vi "Get Timestamp Definition.vi"(11 "Timestamp in":refnum<class "Timestamp.lvclass">) -> (2 "Definition":T1)   [LabVIEW 2020, in "Conditu2.lvlib" / "Columns.lvlib" / "Timestamp.lvclass"]
uses:
  Timestamp.lvclass
  Definition.ctl
  Timestamp.lvclass/Timestamp.ctl
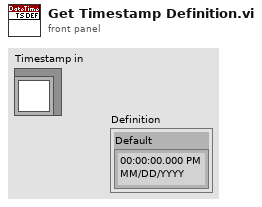
[diagram p1: front panel]
types:
  T1 = typedef "Conditu2.lvlib/Columns.lvlib/Timestamp.lvclass/Definition.ctl" = cluster{"Default":timestamp}
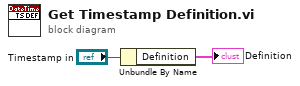
[diagram p0: block diagram]
diagram:
  n1 = Unbundle By Name("Timestamp in") -> ("Definition"=→"Definition":T1)
